vi "fitting express.vi"() -> ()   [LabVIEW 2020]
uses:
  <vilib>/Analysis/NI_AALPro.lvlib
panel:
  out "Niepewnosc 2":dbl
  out "Niepewnosc":dbl
  out "Wielomian najlepszego dopasowania stopnia 5 przy uzyciu express":dbl[][](graph)
  out "Wielomian najlepszego dopasowania stopnia 3 express":dbl[][](graph)
  out "stopnia 5 policzony recznie":dbl[][](graph)
  out "Wielomian najlepszego dopasowania stopnia 3 policzonny recznie":dbl[][](graph)
  in  "k":dbl
  in  "N":i32
  in  "Faza":dbl
  in  "Amplituda":dbl
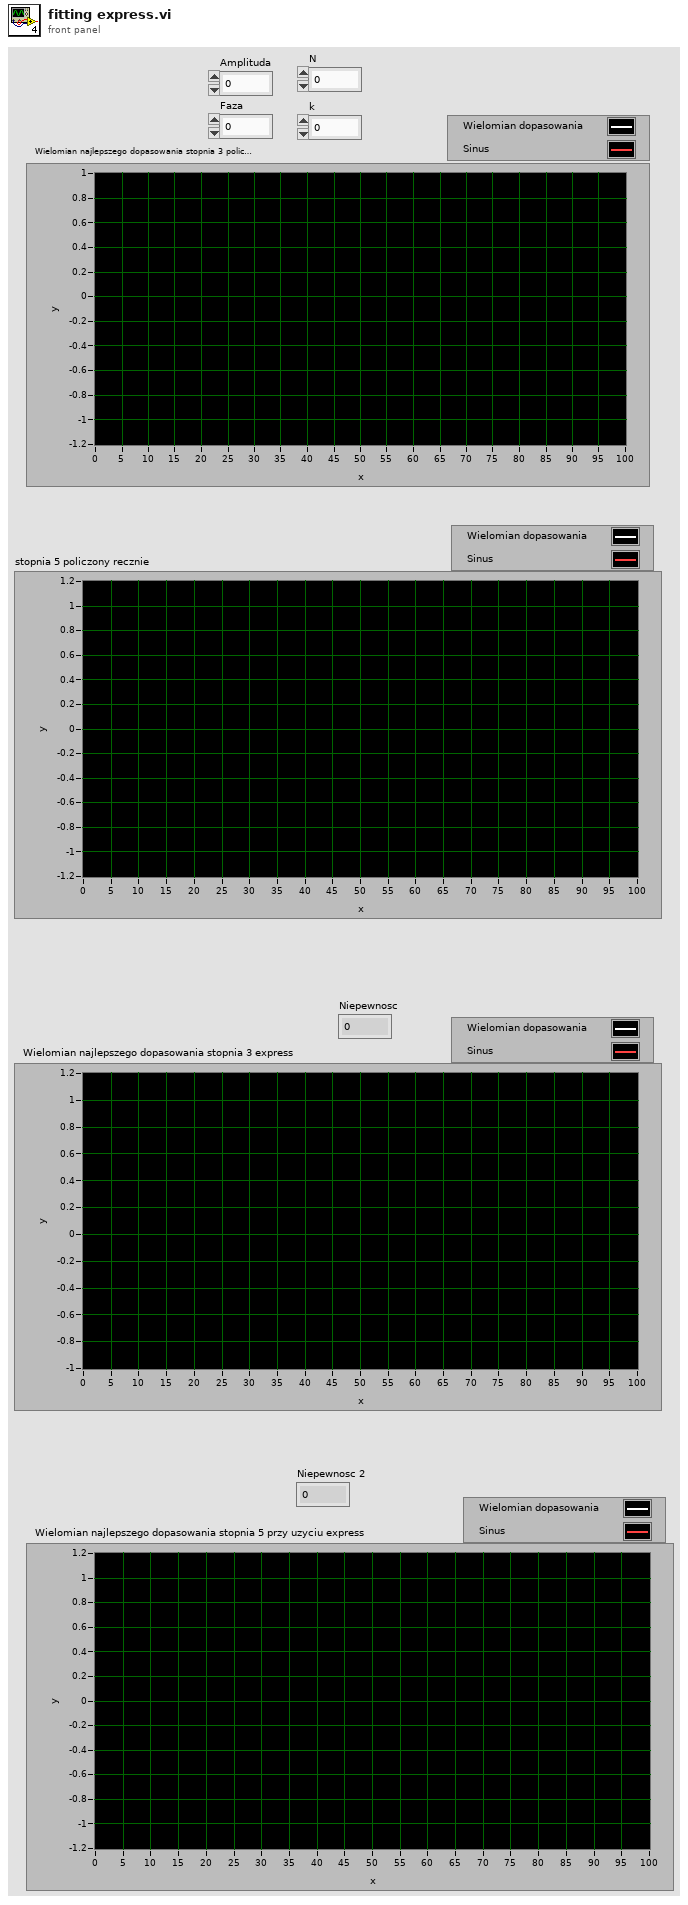
[diagram p1: front panel]
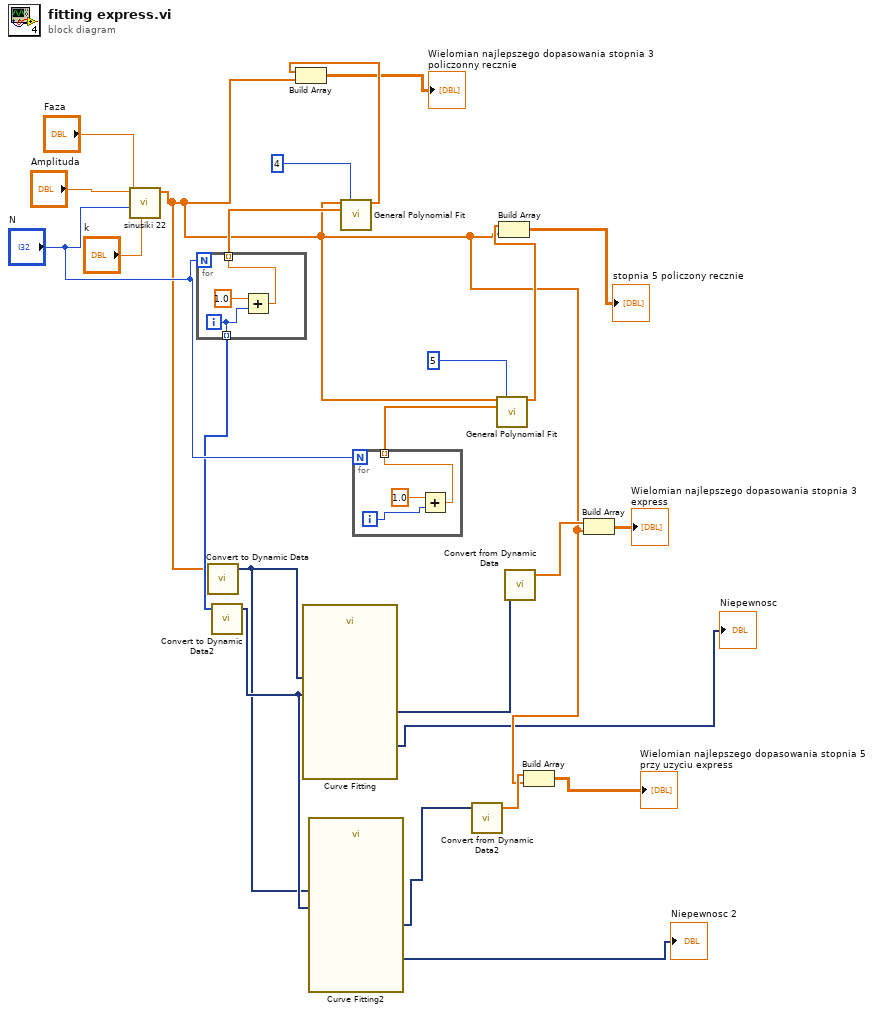
[diagram p0: block diagram]
diagram:
  n1 = call "sinusiki 22.vi"("k"="k", "N"="N", "Faza"="Faza", "Amplituda"="Amplituda") -> ("Array"=w3:dbl[])  [unwired: 7 in]
  n2 = for {
    N: "N" -> [_]
    tunnel: [w26] -> w20 mode=indexing
    tunnel: [w25] -> w11 mode=indexing
    i -> [w25]
    n3 = Add(x=1.0, y=w25) -> (x+y=w26:dbl)
  }
  n4 = call "Convert to Dynamic Data"("Array"=w3) -> ("Dynamic Data Type"=w7:dynamicdata)  [unwired: 3 in]
  n5 = call "Convert to Dynamic Data2"("Array"=w11) -> ("Dynamic Data Type"=w8:dynamicdata)  [unwired: 3 in]
  n6 = call "Curve Fitting"("Locations"=w8, "Signals"=w7) -> ("mean squared error"=→"Niepewnosc":dynamicdata, "best fit"=w13:dynamicdata)  [unwired: 5 in, 3 out]
  n7 = call "Curve Fitting2"("Locations"=w8, "Signals"=w7) -> ("mean squared error"=→"Niepewnosc 2":dynamicdata, "best fit"=w6:dynamicdata)  [unwired: 5 in, 3 out]
  n8 = call <vilib>:"General Polynomial Fit.vi"("Y"=w3, "polynomial order"=4, "X"=w20) -> ("Best Polynomial Fit"=w17:dbl[])  [unwired: 9 in, 3 out]
  n9 = Build Array(w17, w3) -> (→"Wielomian najlepszego dopasowania stopnia 3 policzonny recznie":dbl[][])
  n10 = for {
    N: "N" -> [_]
    tunnel: [w28] -> w18 mode=indexing
    i -> [w29]
    n11 = Add(x=1.0, y=w29) -> (x+y=w28:dbl)
  }
  n12 = call "Convert from Dynamic Data2"("Dynamic Data Type"=w6) -> ("Array"=w5:dbl[])  [unwired: 3 in]
  n13 = call <vilib>:"General Polynomial Fit.vi"("Y"=w3, "polynomial order"=5, "X"=w18) -> ("Best Polynomial Fit"=w14:dbl[])  [unwired: 9 in, 3 out]
  n14 = Build Array(w14, w3) -> (→"stopnia 5 policzony recznie":dbl[][])
  n15 = call "Convert from Dynamic Data"("Dynamic Data Type"=w13) -> ("Array"=w9:dbl[])  [unwired: 3 in]
  n16 = Build Array(w5, w3) -> (→"Wielomian najlepszego dopasowania stopnia 5 przy uzyciu express":dbl[][])
  n17 = Build Array(w9, w3) -> (→"Wielomian najlepszego dopasowania stopnia 3 express":dbl[][])
